vi "Feature_whole(SubVI).vi"(0 "Binary Image":T1) -> (4 "SE":dbl, 5 "rgb Hull Image 2":T1(plugin-control), 6 "SA":dbl, 7 "bw Hull Image 2":T1(plugin-control), 8 "SFD":sgl, 9 "Hull area":dbl, 10 "SW":dbl, 11 "SF 2":dbl, 12 "IFD":sgl, 13 "top":i32, 14 "SF":dbl, 15 "SH":dbl)   [LabVIEW 2015]
uses:
  <vilib>/vision/Image Controls.llb/IMAQ Image.ctl
  <vilib>/vision/NI_Vision_Development_Module.lvlib
  2-top_features_oilseed/fractaldim.dll
  TotalContoursConvexHull.dll
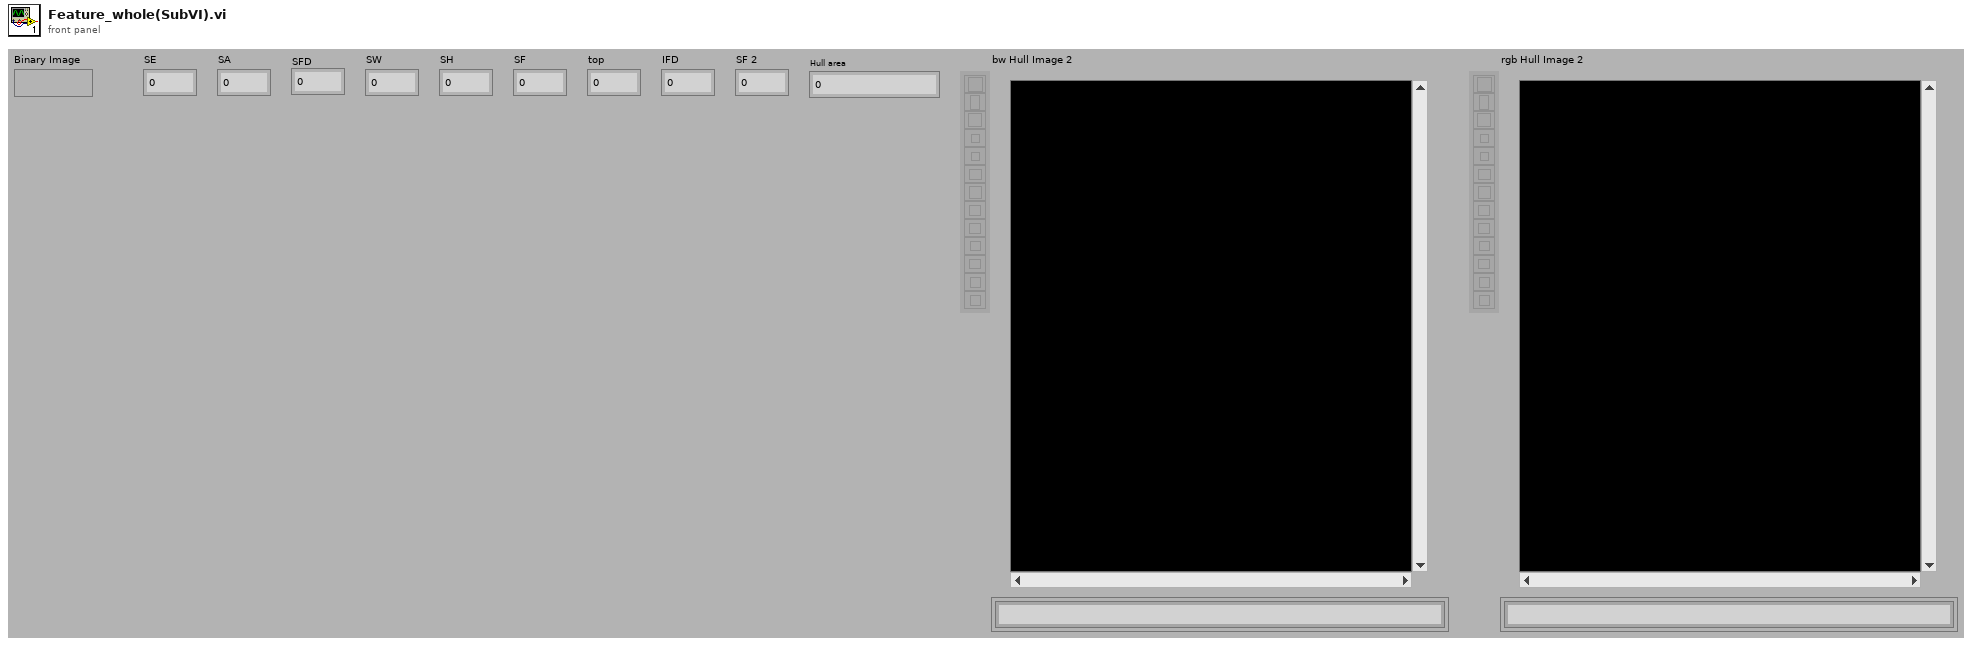
[diagram p1: front panel]
types:
  T1 = typedef "IMAQ Image.ctl" = refnum<image>
  T2 = typedef "Particle Parameters" = i32
  T3 = typedef "Image Type" = u32
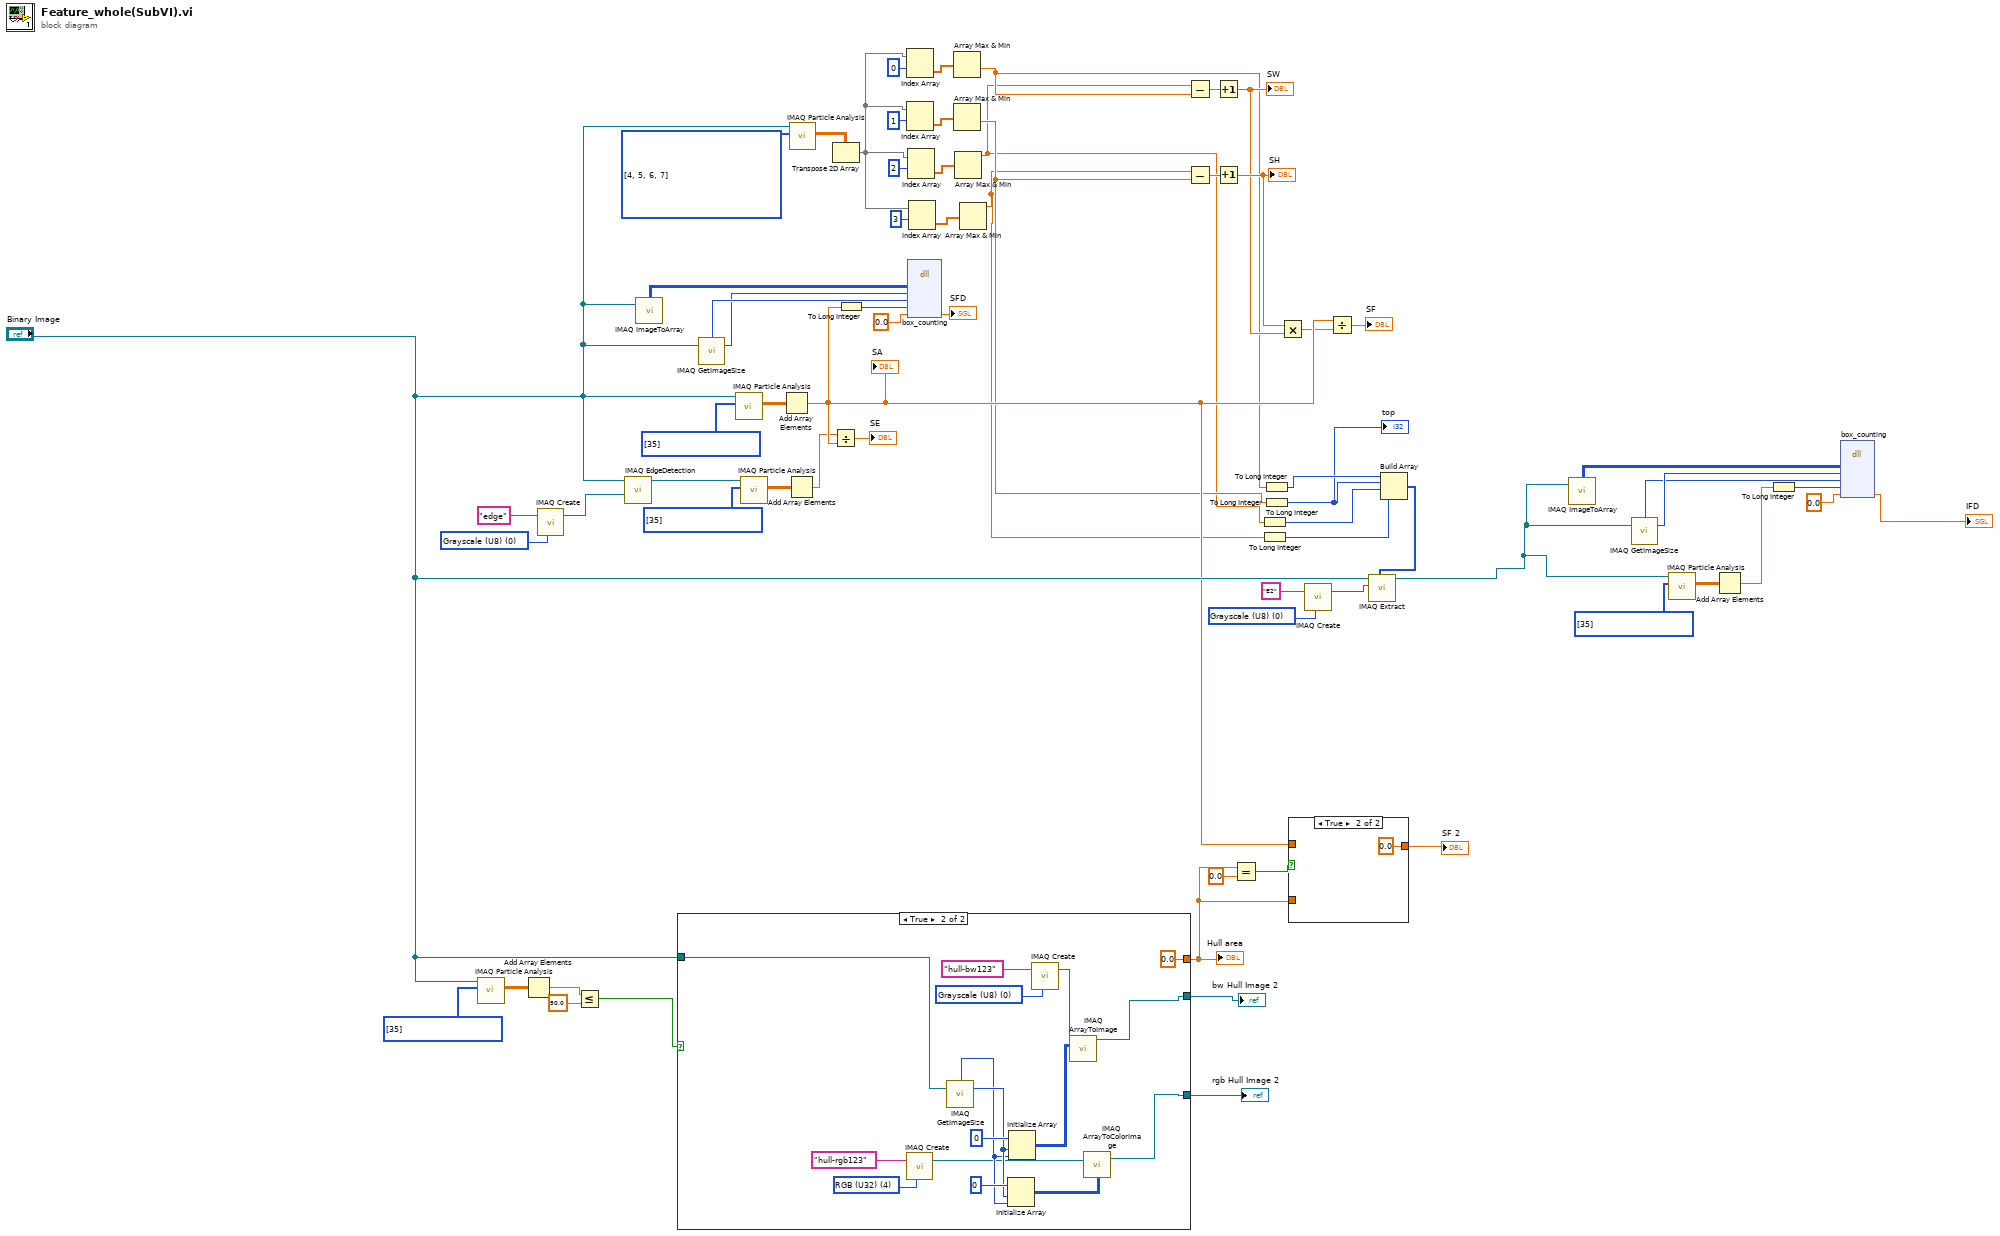
[diagram p0: block diagram]
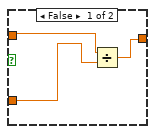
[diagram p2: hidden frame]
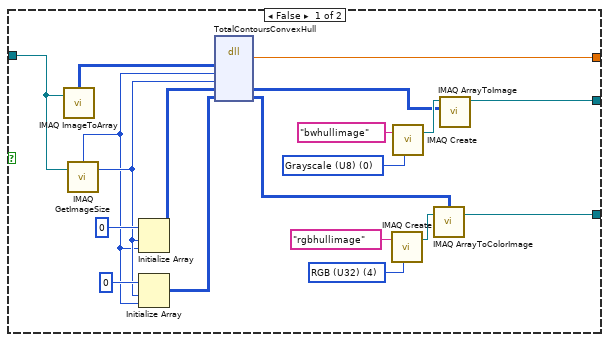
[diagram p3: hidden frame]
diagram:
  w3 = T2[] [35] items=["Center of Mass X", "Center of Mass Y", "First Pixel X", "First Pixel Y", "Bounding Rect Left", "Bounding Rect Top", "Bounding Rect Right", "Bounding Rect Bottom", "Max Feret Diameter Start X", "Max Feret Diameter Start Y", "Max Feret Diameter End X", "Max Feret Diameter End Y", "Max Horiz. Segment Length Left", "Max Horiz. Segment Length Right", "Max Horiz. Segment Length Row", "-", "Bounding Rect Width", "Bounding Rect Height", "Bounding Rect Diagonal", "Perimeter", "Convex Hull Perimeter", "Holes' Perimeter", "Max Feret Diameter", "Equivalent Ellipse Major Axis", "Equivalent Ellipse Minor Axis", "Equivalent Ellipse Minor Axis (Feret)", "Equivalent Rect Long Side", "Equivalent Rect Short Side", "Equivalent Rect Diagonal", "Equivalent Rect Short Side (Feret)", "Average Horiz. Segment Length", "Average Vert. Segment Length", "Hydraulic Radius", "Waddel Disk Diameter", "-", "Area", "Holes' Area", "Particle & Holes' Area", "Convex Hull Area", "Image Area", "-", "Number of Holes", "Number of Horiz. Segments", "Number of Vert. Segments", "-", "Orientation", "Max Feret Diameter Orientation", "-", "% Area/Image Area", "% Area/(Particle & Holes' Area)", "Ratio of Equivalent Ellipse Axes", "Ratio of Equivalent Rect Sides", "-", "Elongation Factor", "Compactness Factor", "Heywood Circularity Factor", "Type Factor", "-", "Sum X", "Sum Y", "Sum XX", "Sum XY", "Sum YY", "Sum XXX", "Sum XXY", "Sum XYY", "Sum YYY", "-", "Moment of Inertia XX", "Moment of Inertia XY", "Moment of Inertia YY", "Moment of Inertia XXX", "Moment of Inertia XXY", "Moment of Inertia XYY", "Moment of Inertia YYY", "Norm. Moment of Inertia XX", "Norm. Moment of Inertia XY", "Norm. Moment of Inertia YY", "Norm. Moment of Inertia XXX", "Norm. Moment of Inertia XXY", "Norm. Moment of Inertia XYY", "Norm. Moment of Inertia YYY", "Hu Moment 1", "Hu Moment 2", "Hu Moment 3", "Hu Moment 4", "Hu Moment 5", "Hu Moment 6", "Hu Moment 7"] ("Pixel Measurements")
  w56 = T2[] [35] items=["Center of Mass X", "Center of Mass Y", "First Pixel X", "First Pixel Y", "Bounding Rect Left", "Bounding Rect Top", "Bounding Rect Right", "Bounding Rect Bottom", "Max Feret Diameter Start X", "Max Feret Diameter Start Y", "Max Feret Diameter End X", "Max Feret Diameter End Y", "Max Horiz. Segment Length Left", "Max Horiz. Segment Length Right", "Max Horiz. Segment Length Row", "-", "Bounding Rect Width", "Bounding Rect Height", "Bounding Rect Diagonal", "Perimeter", "Convex Hull Perimeter", "Holes' Perimeter", "Max Feret Diameter", "Equivalent Ellipse Major Axis", "Equivalent Ellipse Minor Axis", "Equivalent Ellipse Minor Axis (Feret)", "Equivalent Rect Long Side", "Equivalent Rect Short Side", "Equivalent Rect Diagonal", "Equivalent Rect Short Side (Feret)", "Average Horiz. Segment Length", "Average Vert. Segment Length", "Hydraulic Radius", "Waddel Disk Diameter", "-", "Area", "Holes' Area", "Particle & Holes' Area", "Convex Hull Area", "Image Area", "-", "Number of Holes", "Number of Horiz. Segments", "Number of Vert. Segments", "-", "Orientation", "Max Feret Diameter Orientation", "-", "% Area/Image Area", "% Area/(Particle & Holes' Area)", "Ratio of Equivalent Ellipse Axes", "Ratio of Equivalent Rect Sides", "-", "Elongation Factor", "Compactness Factor", "Heywood Circularity Factor", "Type Factor", "-", "Sum X", "Sum Y", "Sum XX", "Sum XY", "Sum YY", "Sum XXX", "Sum XXY", "Sum XYY", "Sum YYY", "-", "Moment of Inertia XX", "Moment of Inertia XY", "Moment of Inertia YY", "Moment of Inertia XXX", "Moment of Inertia XXY", "Moment of Inertia XYY", "Moment of Inertia YYY", "Norm. Moment of Inertia XX", "Norm. Moment of Inertia XY", "Norm. Moment of Inertia YY", "Norm. Moment of Inertia XXX", "Norm. Moment of Inertia XXY", "Norm. Moment of Inertia XYY", "Norm. Moment of Inertia YYY", "Hu Moment 1", "Hu Moment 2", "Hu Moment 3", "Hu Moment 4", "Hu Moment 5", "Hu Moment 6", "Hu Moment 7"] ("Pixel Measurements")
  w22 = T3 0 items=["Grayscale (U8)", "Grayscale (I16)", "Grayscale (SGL)", "Complex (CSG)", "RGB (U32)", "HSL (U32)", "RGB (U64)", "Grayscale (U16)"] ("Image Type")
  w39 = T2[] [4, 5, 6, 7] items=["Center of Mass X", "Center of Mass Y", "First Pixel X", "First Pixel Y", "Bounding Rect Left", "Bounding Rect Top", "Bounding Rect Right", "Bounding Rect Bottom", "Max Feret Diameter Start X", "Max Feret Diameter Start Y", "Max Feret Diameter End X", "Max Feret Diameter End Y", "Max Horiz. Segment Length Left", "Max Horiz. Segment Length Right", "Max Horiz. Segment Length Row", "-", "Bounding Rect Width", "Bounding Rect Height", "Bounding Rect Diagonal", "Perimeter", "Convex Hull Perimeter", "Holes' Perimeter", "Max Feret Diameter", "Equivalent Ellipse Major Axis", "Equivalent Ellipse Minor Axis", "Equivalent Ellipse Minor Axis (Feret)", "Equivalent Rect Long Side", "Equivalent Rect Short Side", "Equivalent Rect Diagonal", "Equivalent Rect Short Side (Feret)", "Average Horiz. Segment Length", "Average Vert. Segment Length", "Hydraulic Radius", "Waddel Disk Diameter", "-", "Area", "Holes' Area", "Particle & Holes' Area", "Convex Hull Area", "Image Area", "-", "Number of Holes", "Number of Horiz. Segments", "Number of Vert. Segments", "-", "Orientation", "Max Feret Diameter Orientation", "-", "% Area/Image Area", "% Area/(Particle & Holes' Area)", "Ratio of Equivalent Ellipse Axes", "Ratio of Equivalent Rect Sides", "-", "Elongation Factor", "Compactness Factor", "Heywood Circularity Factor", "Type Factor", "-", "Sum X", "Sum Y", "Sum XX", "Sum XY", "Sum YY", "Sum XXX", "Sum XXY", "Sum XYY", "Sum YYY", "-", "Moment of Inertia XX", "Moment of Inertia XY", "Moment of Inertia YY", "Moment of Inertia XXX", "Moment of Inertia XXY", "Moment of Inertia XYY", "Moment of Inertia YYY", "Norm. Moment of Inertia XX", "Norm. Moment of Inertia XY", "Norm. Moment of Inertia YY", "Norm. Moment of Inertia XXX", "Norm. Moment of Inertia XXY", "Norm. Moment of Inertia XYY", "Norm. Moment of Inertia YYY", "Hu Moment 1", "Hu Moment 2", "Hu Moment 3", "Hu Moment 4", "Hu Moment 5", "Hu Moment 6", "Hu Moment 7"] ("Pixel Measurements")
  w48 = T2[] [35] items=["Center of Mass X", "Center of Mass Y", "First Pixel X", "First Pixel Y", "Bounding Rect Left", "Bounding Rect Top", "Bounding Rect Right", "Bounding Rect Bottom", "Max Feret Diameter Start X", "Max Feret Diameter Start Y", "Max Feret Diameter End X", "Max Feret Diameter End Y", "Max Horiz. Segment Length Left", "Max Horiz. Segment Length Right", "Max Horiz. Segment Length Row", "-", "Bounding Rect Width", "Bounding Rect Height", "Bounding Rect Diagonal", "Perimeter", "Convex Hull Perimeter", "Holes' Perimeter", "Max Feret Diameter", "Equivalent Ellipse Major Axis", "Equivalent Ellipse Minor Axis", "Equivalent Ellipse Minor Axis (Feret)", "Equivalent Rect Long Side", "Equivalent Rect Short Side", "Equivalent Rect Diagonal", "Equivalent Rect Short Side (Feret)", "Average Horiz. Segment Length", "Average Vert. Segment Length", "Hydraulic Radius", "Waddel Disk Diameter", "-", "Area", "Holes' Area", "Particle & Holes' Area", "Convex Hull Area", "Image Area", "-", "Number of Holes", "Number of Horiz. Segments", "Number of Vert. Segments", "-", "Orientation", "Max Feret Diameter Orientation", "-", "% Area/Image Area", "% Area/(Particle & Holes' Area)", "Ratio of Equivalent Ellipse Axes", "Ratio of Equivalent Rect Sides", "-", "Elongation Factor", "Compactness Factor", "Heywood Circularity Factor", "Type Factor", "-", "Sum X", "Sum Y", "Sum XX", "Sum XY", "Sum YY", "Sum XXX", "Sum XXY", "Sum XYY", "Sum YYY", "-", "Moment of Inertia XX", "Moment of Inertia XY", "Moment of Inertia YY", "Moment of Inertia XXX", "Moment of Inertia XXY", "Moment of Inertia XYY", "Moment of Inertia YYY", "Norm. Moment of Inertia XX", "Norm. Moment of Inertia XY", "Norm. Moment of Inertia YY", "Norm. Moment of Inertia XXX", "Norm. Moment of Inertia XXY", "Norm. Moment of Inertia XYY", "Norm. Moment of Inertia YYY", "Hu Moment 1", "Hu Moment 2", "Hu Moment 3", "Hu Moment 4", "Hu Moment 5", "Hu Moment 6", "Hu Moment 7"] ("Pixel Measurements")
  w51 = T3 0 items=["Grayscale (U8)", "Grayscale (I16)", "Grayscale (SGL)", "Complex (CSG)", "RGB (U32)", "HSL (U32)", "RGB (U64)", "Grayscale (U16)"] ("Image Type")
  w54 = T2[] [35] items=["Center of Mass X", "Center of Mass Y", "First Pixel X", "First Pixel Y", "Bounding Rect Left", "Bounding Rect Top", "Bounding Rect Right", "Bounding Rect Bottom", "Max Feret Diameter Start X", "Max Feret Diameter Start Y", "Max Feret Diameter End X", "Max Feret Diameter End Y", "Max Horiz. Segment Length Left", "Max Horiz. Segment Length Right", "Max Horiz. Segment Length Row", "-", "Bounding Rect Width", "Bounding Rect Height", "Bounding Rect Diagonal", "Perimeter", "Convex Hull Perimeter", "Holes' Perimeter", "Max Feret Diameter", "Equivalent Ellipse Major Axis", "Equivalent Ellipse Minor Axis", "Equivalent Ellipse Minor Axis (Feret)", "Equivalent Rect Long Side", "Equivalent Rect Short Side", "Equivalent Rect Diagonal", "Equivalent Rect Short Side (Feret)", "Average Horiz. Segment Length", "Average Vert. Segment Length", "Hydraulic Radius", "Waddel Disk Diameter", "-", "Area", "Holes' Area", "Particle & Holes' Area", "Convex Hull Area", "Image Area", "-", "Number of Holes", "Number of Horiz. Segments", "Number of Vert. Segments", "-", "Orientation", "Max Feret Diameter Orientation", "-", "% Area/Image Area", "% Area/(Particle & Holes' Area)", "Ratio of Equivalent Ellipse Axes", "Ratio of Equivalent Rect Sides", "-", "Elongation Factor", "Compactness Factor", "Heywood Circularity Factor", "Type Factor", "-", "Sum X", "Sum Y", "Sum XX", "Sum XY", "Sum YY", "Sum XXX", "Sum XXY", "Sum XYY", "Sum YYY", "-", "Moment of Inertia XX", "Moment of Inertia XY", "Moment of Inertia YY", "Moment of Inertia XXX", "Moment of Inertia XXY", "Moment of Inertia XYY", "Moment of Inertia YYY", "Norm. Moment of Inertia XX", "Norm. Moment of Inertia XY", "Norm. Moment of Inertia YY", "Norm. Moment of Inertia XXX", "Norm. Moment of Inertia XXY", "Norm. Moment of Inertia XYY", "Norm. Moment of Inertia YYY", "Hu Moment 1", "Hu Moment 2", "Hu Moment 3", "Hu Moment 4", "Hu Moment 5", "Hu Moment 6", "Hu Moment 7"] ("Pixel Measurements")
  n1 = call "IMAQ Particle Analysis"("Pixel Measurements"=w56, "Image"="Binary Image") -> ("Particle Measurements (Pixels)"=w57:dbl[][])  [unwired: 3 in, 6 out]
  n2 = Add Array Elements(numeric array=w57) -> (sum=w59:dbl)
  n3 = call "IMAQ Create"("Image Name"="edge", "Image Type"=w51) -> ("New Image"=w50:T1)  [unwired: 2 in, 2 out]
  n4 = Less Or Equal?(x=w59, y=50.0) -> (x <= y?=w60:bool)
  n5 = call "IMAQ EdgeDetection"("Image Dst"=w50, "Image Src"="Binary Image") -> ("Image Dst Out"=w53:T1)  [unwired: 4 in, 5 out]
  n6 = call "IMAQ ImageToArray"("Image"="Binary Image") -> ("Image Pixels (U8)"=w44:u8[][])  [unwired: 2 in, 5 out]
  n7 = case shown="True" w60 {
    tunnel: "Binary Image" -> [w72 w101]
    tunnel: [w71 0.0 ("areaSum")] -> w65
    tunnel: [w70 w99] -> w66
    tunnel: [w69 w88] -> w67
    frame False {
      w75 = T3 4 items=["Grayscale (U8)", "Grayscale (I16)", "Grayscale (SGL)", "Complex (CSG)", "RGB (U32)", "HSL (U32)", "RGB (U64)", "Grayscale (U16)"] ("Image Type")
      w85 = T3 0 items=["Grayscale (U8)", "Grayscale (I16)", "Grayscale (SGL)", "Complex (CSG)", "RGB (U32)", "HSL (U32)", "RGB (U64)", "Grayscale (U16)"] ("Image Type")
      n8 = call "IMAQ ImageToArray"("Image"=w72) -> ("Image Pixels (U8)"=w87:u8[][])  [unwired: 2 in, 5 out]
      n9 = call "IMAQ GetImageSize"("Image"=w72) -> ("Y Resolution"=w78:i32, "X Resolution"=w77:i32)  [unwired: 1 in, 3 out]
      n10 = Initialize Array(u8 0 ("element"), w78, w77) -> (w83:u8[][])
      n11 = Initialize Array(u32 0 ("element"), w78, w77) -> (w79:u32[][])
      n12 = dll-call lib="H:/3-side_features_oilseed/TotalContoursConvexHull.dll" fn="TotalContoursConvexHull"("src"=w87, "width"=w77, "height"=w78, "bwhullimage"=w83, "rgbhullimage"=w79) -> ("areaSum"=w71:dbl, "bwhullimage"=w81:u8[][], "rgbhullimage"=w74:u32[][])  [unwired: 6 in, 2 out]
      n13 = call "IMAQ Create"("Image Name"="rgbhullimage", "Image Type"=w75) -> ("New Image"=w73:T1)  [unwired: 2 in, 2 out]
      n14 = call "IMAQ Create"("Image Name"="bwhullimage", "Image Type"=w85) -> ("New Image"=w84:T1)  [unwired: 2 in, 2 out]
      n15 = call "IMAQ ArrayToColorImage"("Image Pixels (U32)"=w74, "Image"=w73) -> ("Image Out"=w69:T1)  [unwired: 2 in, 2 out]
      n16 = call "IMAQ ArrayToImage"("Image Pixels (U8)"=w81, "Image"=w84) -> ("Image Out"=w70:T1)  [unwired: 4 in, 5 out]
    }
    frame True {
      w90 = T3 4 items=["Grayscale (U8)", "Grayscale (I16)", "Grayscale (SGL)", "Complex (CSG)", "RGB (U32)", "HSL (U32)", "RGB (U64)", "Grayscale (U16)"] ("Image Type")
      w98 = T3 0 items=["Grayscale (U8)", "Grayscale (I16)", "Grayscale (SGL)", "Complex (CSG)", "RGB (U32)", "HSL (U32)", "RGB (U64)", "Grayscale (U16)"] ("Image Type")
      n17 = call "IMAQ Create"("Image Name"="hull-rgb123", "Image Type"=w90) -> ("New Image"=w89:T1)  [unwired: 2 in, 2 out]
      n18 = call "IMAQ GetImageSize"("Image"=w101) -> ("Y Resolution"=w94:i32, "X Resolution"=w93:i32)  [unwired: 1 in, 3 out]
      n19 = Initialize Array(u32 0 ("element"), w94, w93) -> (w92:u32[][])
      n20 = Initialize Array(u8 0 ("element"), w94, w93) -> (w100:u8[][])
      n21 = call "IMAQ Create"("Image Name"="hull-bw123", "Image Type"=w98) -> ("New Image"=w96:T1)  [unwired: 2 in, 2 out]
      n22 = call "IMAQ ArrayToImage"("Image Pixels (U8)"=w100, "Image"=w96) -> ("Image Out"=w99:T1)  [unwired: 4 in, 5 out]
      n23 = call "IMAQ ArrayToColorImage"("Image Pixels (U32)"=w92, "Image"=w89) -> ("Image Out"=w88:T1)  [unwired: 2 in, 2 out]
    }
  }
  "Hull area" <- w65
  "bw Hull Image 2" <- w66
  "rgb Hull Image 2" <- w67
  n24 = call "IMAQ GetImageSize"("Image"="Binary Image") -> ("Y Resolution"=w40:i32, "X Resolution"=w41:i32)  [unwired: 1 in, 3 out]
  n25 = call "IMAQ Particle Analysis"("Pixel Measurements"=w48, "Image"="Binary Image") -> ("Particle Measurements (Pixels)"=w49:dbl[][])  [unwired: 3 in, 6 out]
  n26 = call "IMAQ Particle Analysis"("Pixel Measurements"=w54, "Image"=w53) -> ("Particle Measurements (Pixels)"=w55:dbl[][])  [unwired: 3 in, 6 out]
  n27 = Add Array Elements(numeric array=w49) -> (sum=w63:dbl)
  "SA" <- w63
  n28 = Add Array Elements(numeric array=w55) -> (sum=w47:dbl)
  n29 = call "IMAQ Particle Analysis"("Pixel Measurements"=w39, "Image"="Binary Image") -> ("Particle Measurements (Pixels)"=w38:dbl[][])  [unwired: 3 in, 6 out]
  n30 = Transpose 2D Array(2D array=w38) -> (transposed array=w29:dbl[][])
  n31 = Divide(x=w47, y=w63) -> (x/y=→"SE":dbl)
  n32 = To Long Integer(number=w63) -> (32bit integer=w43:i32)
  n33 = Index Array(array=w29, index (row)=0) -> (element=w31:dbl[])  [unwired: 1 in]
  n34 = Index Array(array=w29, index (row)=1) -> (element=w32:dbl[])  [unwired: 1 in]
  n35 = Index Array(array=w29, index (row)=2) -> (element=w36:dbl[])  [unwired: 1 in]
  n36 = dll-call lib="H:/2-top_features_oilseed/fractaldim.dll" fn="box_counting"("bw"=w44, "row"=w40, "col"=w41, "area"=w43, "FD"=sgl 0.0) -> ("FD"=→"SFD":sgl)  [unwired: 7 in, 3 out]
  n37 = Index Array(array=w29, index (row)=3) -> (element=w35:dbl[])  [unwired: 1 in]
  n38 = Array Max & Min(array=w31) -> (min value=w19:dbl)  [unwired: 3 out]
  n39 = Array Max & Min(array=w32) -> (min value=w17:dbl)  [unwired: 3 out]
  n40 = Array Max & Min(array=w36) -> (max value=w15:dbl)  [unwired: 3 out]
  n41 = Array Max & Min(array=w35) -> (max value=w13:dbl)  [unwired: 3 out]
  n42 = Subtract(x=w15, y=w19) -> (x-y=w28:dbl)
  n43 = Subtract(x=w13, y=w17) -> (x-y=w27:dbl)
  n44 = Increment(x=w28) -> (x+1=w24:dbl)
  "SW" <- w24
  n45 = Increment(x=w27) -> (x+1=w25:dbl)
  "SH" <- w25
  n46 = Equal?(x=w65, y=0.0) -> (x = y?=w62:bool)
  n47 = To Long Integer(number=w15) -> (32bit integer=w14:i32)
  n48 = To Long Integer(number=w13) -> (32bit integer=w12:i32)
  n49 = To Long Integer(number=w19) -> (32bit integer=w18:i32)
  n50 = To Long Integer(number=w17) -> (32bit integer=w16:i32)
  "top" <- w16
  n51 = Multiply(x=w25, y=w24) -> (x*y=w26:dbl)
  n52 = case shown="True" w62 {
    tunnel: w63 -> [w106 _]
    tunnel: w65 -> [w105 _]
    tunnel: [w104 0.0] -> w64
    frame False {
      n53 = Divide(x=w106, y=w105) -> (x/y=w104:dbl)
    }
    frame True {
    }
  }
  "SF 2" <- w64
  n54 = call "IMAQ Create"("Image Name"="E2", "Image Type"=w22) -> ("New Image"=w20:T1)  [unwired: 2 in, 2 out]
  n55 = Divide(x=w63, y=w26) -> (x/y=→"SF":dbl)
  n56 = Build Array(w18, w16, w14, w12) -> (w11:i32[])
  n57 = call "IMAQ Extract"("Optional Rectangle"=w11, "Image Dst"=w20, "Image Src"="Binary Image") -> ("Image Dst Out"=w10:T1)  [unwired: 3 in, 5 out]
  n58 = call "IMAQ ImageToArray"("Image"=w10) -> ("Image Pixels (U8)"=w5:u8[][])  [unwired: 2 in, 5 out]
  n59 = call "IMAQ GetImageSize"("Image"=w10) -> ("Y Resolution"=w8:i32, "X Resolution"=w7:i32)  [unwired: 1 in, 3 out]
  n60 = call "IMAQ Particle Analysis"("Pixel Measurements"=w3, "Image"=w10) -> ("Particle Measurements (Pixels)"=w2:dbl[][])  [unwired: 3 in, 6 out]
  n61 = Add Array Elements(numeric array=w2) -> (sum=w9:dbl)
  n62 = To Long Integer(number=w9) -> (32bit integer=w6:i32)
  n63 = dll-call lib="H:/2-top_features_oilseed/fractaldim.dll" fn="box_counting"("bw"=w5, "row"=w8, "col"=w7, "area"=w6, "FD"=sgl 0.0) -> ("FD"=→"IFD":sgl)  [unwired: 7 in, 3 out]
